vi "FPGA Initialise.vi"(8 "error in (no error)":errorcluster) -> (0 "error out":errorcluster)   [LabVIEW 2017]
doc: "This VI initialises the FPGA and loads the bit file."
uses:
  <vilib>/FPGAPlugInAG/myRIO-1900/niLvFpga_Open_myRIO-1900.vi
  <vilib>/rvi/interface/common/dynamic/niFpgaDynamicAddResources.vi
  <vilib>/FPGAPlugInAG/Dynamic/niLvFpga_Reset_Dynamic.vi
  <vilib>/FPGAPlugInAG/Dynamic/niLvFpga_Run_Dynamic.vi
  FPGA Global Variables.vi
  <vilib>/rvi/interface/nirviOpenFPGA/nirviOpenFPGA.xnode
  FPGA Bitfiles/MySDRio_FPGATarget_FPGAMain_RLtJEVrxekk.lvbitx
  FPGA/FPGA_Main.vi
  <vilib>/rvi/interface/nirviMethod/nirviMethod.xnode
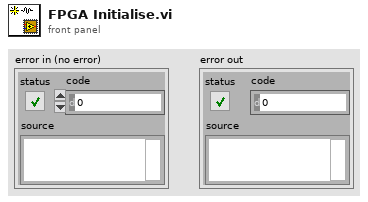
[diagram p1: front panel]
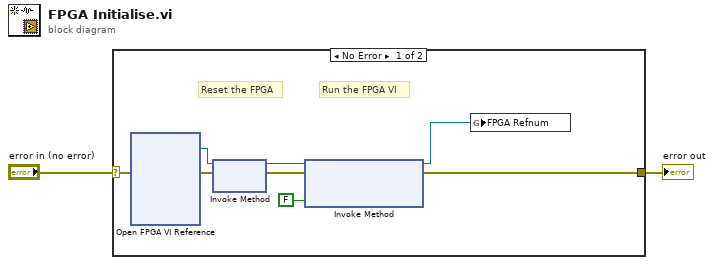
[diagram p0: block diagram]
diagram:
  n1 = case shown="No Error" "error in (no error)" {
    selector: "error in (no error)" -> [w4 w11]
    tunnel: [w10 w11] -> w2
    frame No Error {
      # "Run the FPGA VI"
      # "Reset the FPGA"
      n2 = xnode "Open FPGA VI Reference"("error in"=w4) -> ("FPGA VI Reference Out"=w5:refnum<k20>, "error out"=w6:errorcluster)  [unwired: 1 in]
      n3 = xnode "Invoke Method"("FPGA VI Reference In"=w5, "error in"=w6) -> ("FPGA VI Reference Out"=w7:refnum<k20>, "error out"=w8:errorcluster)
      n4 = xnode "Invoke Method"("FPGA VI Reference In"=w7, "error in"=w8, "Wait Until Done (F)"=FALSE) -> ("FPGA VI Reference Out"=w3:refnum<k20>, "error out"=w10:errorcluster)
      n5 = global write "FPGA Global Variables.vi" "FPGA Refnum"(w3) -> ()
    }
    frame Error {
    }
  }
  "error out" <- w2
